vi "Artikeldaten_laden.vi"(8 "Fehler in":errorcluster, 11 "Cluster in":T1={"Initialisierung"={"Online?"=FALSE, "Grundpfad"=path "", "Kamera Oben"="", "IP-Adresse Flüssiglinse"="", "Flüssiglinse"=refnum, "Kamera Unten"="", "IP-Adresse SPS"="", "SPS-Verbindung"={"TCP Connection Ref"=refnum, "IP address"="", "timeout ms"=5000, "Connected?"=FALSE, "PLC Type"=enum."S7 1200", "Rack S7 400"=0, "Slot S7 400"=0, "PDU Size"=0, "connection semaphore"=refnum}, "IP-Adresse Lichtgitter"="", "Lichtgitter"=refnum, "Skalierungsfaktor"=0.0, "Bilder Oben"=[], "Bild Unten"=refnum, "Bild Ausschnitt Unten"=refnum}, "Einstellungen"={"Gesamtablauf gestartet"=FALSE, "i. O. Bilder speichern"=FALSE, "Bildspeicherung Offline"=FALSE, "Ausgewähltes Offline-Datum"="", "Ausgewähltes Offline-Teil"="", "Speicherpfad Bilder"=path ""}, "Artikeldaten"={"Artikelnummer"="", "Fertigungsauftrag"="", "Muster ISO"=refnum, "Belichtungszeit Referenzmarken"=0.0, "Fokus Referenzmarken"=0.0, "Belichtungszeit ISO"=0.0, "Fokus ISO"=0.0, "Belichtungszeit Unten"=0.0, "Kontaktanzahl"=0, "Aktueller Kontakt"=0, "Kontaktposition"={"x"=0.0, "y"=0.0}, "ISO-Muster nicht vorhanden"=FALSE, "Winkel ISO"=0.0, "Mittelpunkt ISO"={"x"=0.0, "y"=0.0}}, "Werte Kamera Oben"={"Koordinatensystem"={"Punkt x-Achse"={"X"=0.0, "Y"=0.0}, "Ursprung"={"X"=0.0, "Y"=0.0}, "Punkt y-Achse"={"X"=0.0, "Y"=0.0}}, "Position Kontakt"={"x"=0.0, "y"=0.0}, "Durchmesser Loch"=0.0, "Winkel Kontakt"=0.0, "Position Kontakt umgerechnet"={"x"=0.0, "y"=0.0}}, "Werte Kamera Unten"={"Prüfung Unten n. i. O."=FALSE}, "Werte Lichtgitter"={"Messwerte Referenzmarken"=[], "Mittelpunkt Referenzmarken"={"x"=0.0, "y"=0.0}, "Messwerte Kontakt"=[], "Offset"={"x"=0.0, "y"=0.0}}, "Rückmeldungen"={"Koordinaten ermittelt"=FALSE, "Vermessung Lichtgitter fertig"=FALSE, "Nachkontrolle Kamera Unten fertig"=FALSE}, "Fehler"={"Referenzen nicht gefunden"=FALSE, "Kontakt nicht gefunden"=FALSE, "Referenzen nicht in Lichtgitter"=FALSE, "Kontakt zu groß"=FALSE, "Kontakt zu klein"=FALSE}, "Statistik"={"Statistiken"=[]}, "Timer"={"Timer Start Position"=0, "Timer Start Lichtgitter"=0, "Timer Start Kamera Unten"=0}}) -> (0 "Fehler out":errorcluster, 1 "Anzahl Bilder out":i32, 2 "Offline Teile-Datum out":string[](array[string]), 3 "Cluster out":T1={"Initialisierung"={"Online?"=FALSE, "Grundpfad"=path "", "Kamera Oben"="", "IP-Adresse Flüssiglinse"="", "Flüssiglinse"=refnum, "Kamera Unten"="", "IP-Adresse SPS"="", "SPS-Verbindung"={"TCP Connection Ref"=refnum, "IP address"="", "timeout ms"=5000, "Connected?"=FALSE, "PLC Type"=enum."S7 1200", "Rack S7 400"=0, "Slot S7 400"=0, "PDU Size"=0, "connection semaphore"=refnum}, "IP-Adresse Lichtgitter"="", "Lichtgitter"=refnum, "Skalierungsfaktor"=0.0, "Bilder Oben"=[], "Bild Unten"=refnum, "Bild Ausschnitt Unten"=refnum}, "Einstellungen"={"Gesamtablauf gestartet"=FALSE, "i. O. Bilder speichern"=FALSE, "Bildspeicherung Offline"=FALSE, "Ausgewähltes Offline-Datum"="", "Ausgewähltes Offline-Teil"="", "Speicherpfad Bilder"=path ""}, "Artikeldaten"={"Artikelnummer"="", "Fertigungsauftrag"="", "Muster ISO"=refnum, "Belichtungszeit Referenzmarken"=0.0, "Fokus Referenzmarken"=0.0, "Belichtungszeit ISO"=0.0, "Fokus ISO"=0.0, "Belichtungszeit Unten"=0.0, "Kontaktanzahl"=0, "Aktueller Kontakt"=0, "Kontaktposition"={"x"=0.0, "y"=0.0}, "ISO-Muster nicht vorhanden"=FALSE, "Winkel ISO"=0.0, "Mittelpunkt ISO"={"x"=0.0, "y"=0.0}}, "Werte Kamera Oben"={"Koordinatensystem"={"Punkt x-Achse"={"X"=0.0, "Y"=0.0}, "Ursprung"={"X"=0.0, "Y"=0.0}, "Punkt y-Achse"={"X"=0.0, "Y"=0.0}}, "Position Kontakt"={"x"=0.0, "y"=0.0}, "Durchmesser Loch"=0.0, "Winkel Kontakt"=0.0, "Position Kontakt umgerechnet"={"x"=0.0, "y"=0.0}}, "Werte Kamera Unten"={"Prüfung Unten n. i. O."=FALSE}, "Werte Lichtgitter"={"Messwerte Referenzmarken"=[], "Mittelpunkt Referenzmarken"={"x"=0.0, "y"=0.0}, "Messwerte Kontakt"=[], "Offset"={"x"=0.0, "y"=0.0}}, "Rückmeldungen"={"Koordinaten ermittelt"=FALSE, "Vermessung Lichtgitter fertig"=FALSE, "Nachkontrolle Kamera Unten fertig"=FALSE}, "Fehler"={"Referenzen nicht gefunden"=FALSE, "Kontakt nicht gefunden"=FALSE, "Referenzen nicht in Lichtgitter"=FALSE, "Kontakt zu groß"=FALSE, "Kontakt zu klein"=FALSE}, "Statistik"={"Statistiken"=[]}, "Timer"={"Timer Start Position"=0, "Timer Start Lichtgitter"=0, "Timer Start Kamera Unten"=0}})   [LabVIEW 2024]
doc: "Lädt die Artikeldaten aus den Globalen Variablen, bzw. im \"Offline-Modus\" aus der Konfig Datei in das Cluster."
uses:
  Typdefinitionen/Cluster.ctl
  <vilib>/userDefined/High Color/IMAQdx.ctl
  <vilib>/DATA AHEAD/SP7/typedefs/S7 Connection.ctl
  <vilib>/DATA AHEAD/SP7/typedefs/PLC Type.ctl
  <vilib>/vision/Image Controls.llb/IMAQ Image.ctl
  Typdefinitionen/Koordinatensystem.ctl
  Typdefinitionen/Statistik.ctl
  <vilib>/Utility/config.llb/Read Key (U32).vi
  <vilib>/Utility/config.llb/Read Key (Double).vi
  Sonstige/Globale Variablen.vi
  <vilib>/Utility/config.llb/Write Key (U32).vi
  <vilib>/Utility/config.llb/Write Key (Double).vi
  <vilib>/Utility/config.llb/NI_LVConfig.lvlib
  <vilib>/DATA AHEAD/SP7/SP7.lvlib
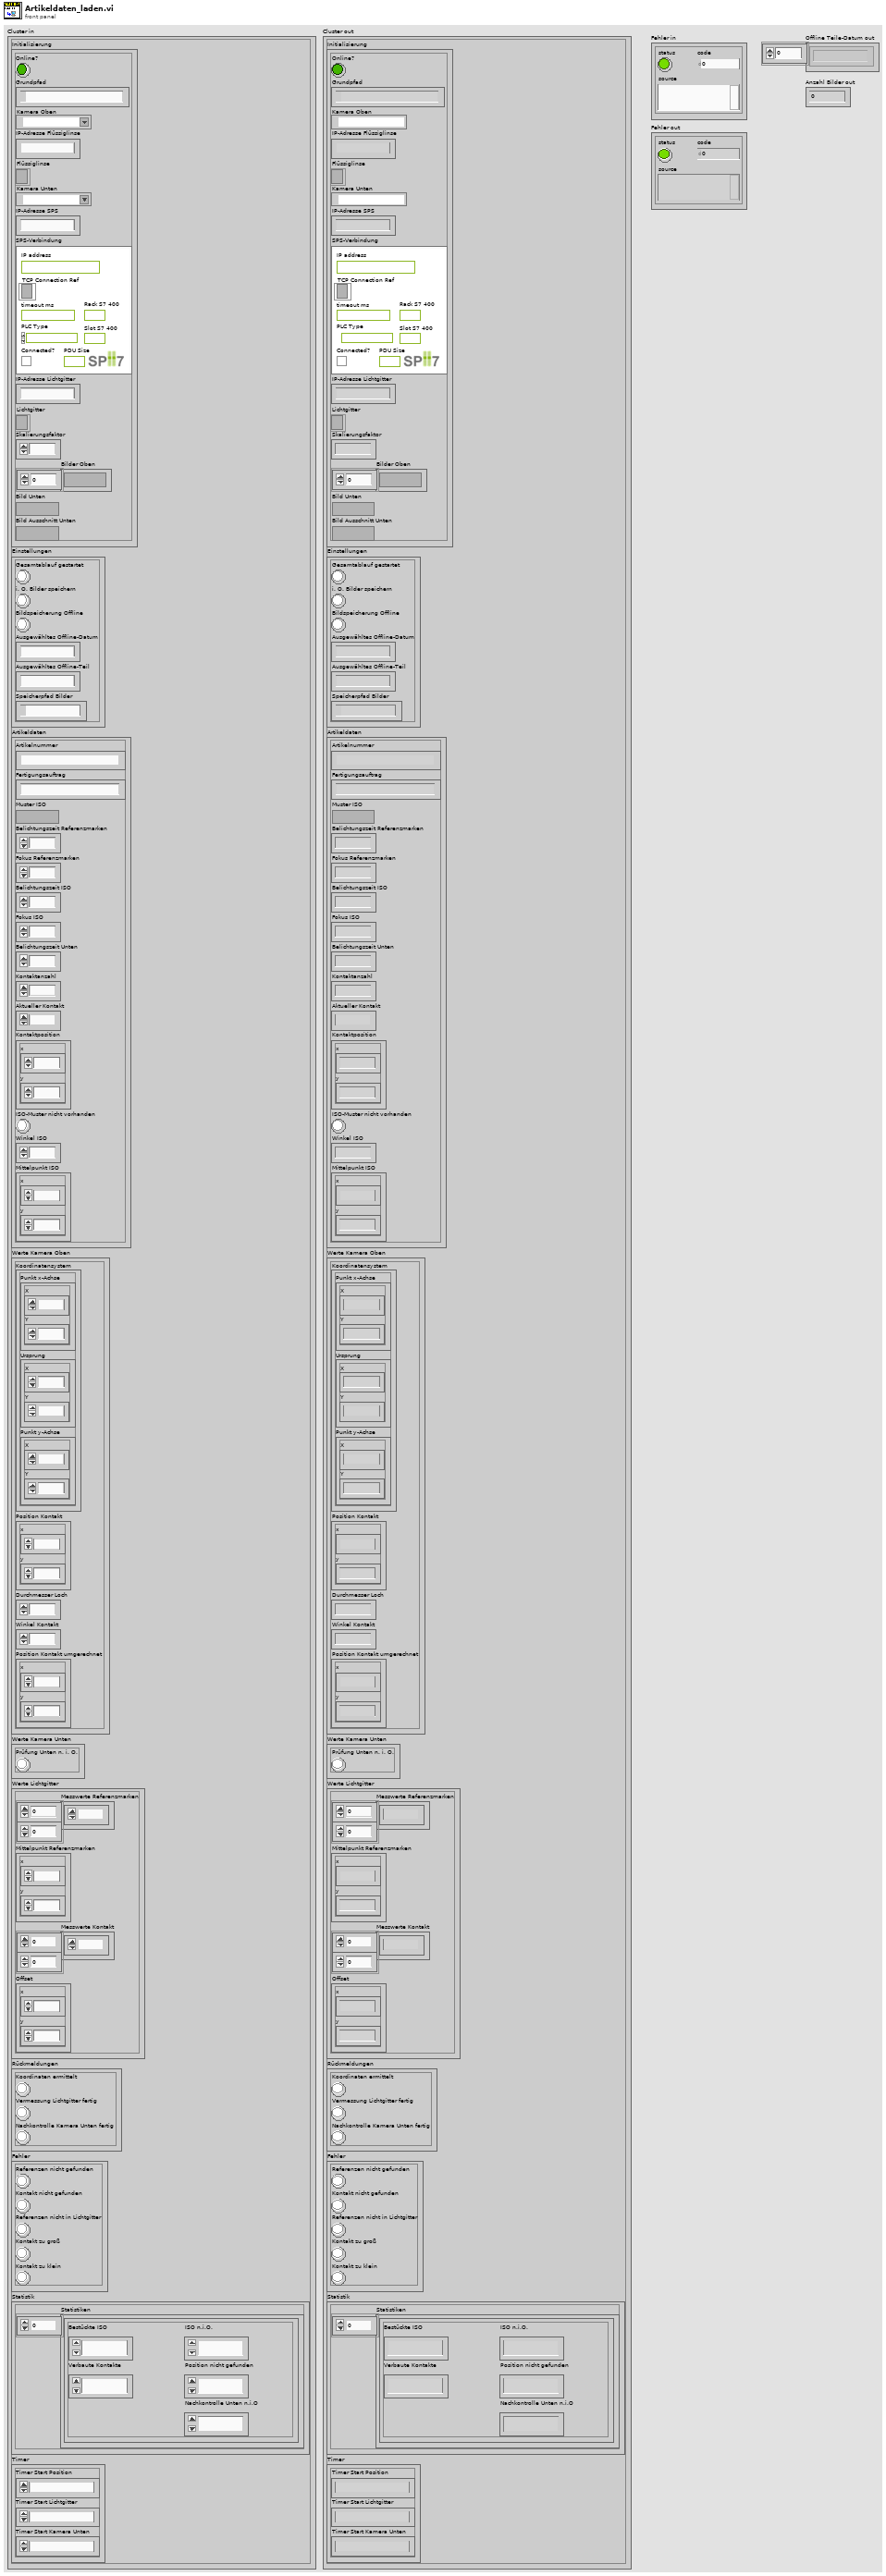
[diagram p1: front panel]
types:
  T1 = typedef "Cluster.ctl" = cluster{"Initialisierung":cluster{"Online?":bool, "Grundpfad":path, "Kamera Oben":T2, "IP-Adresse Flüssiglinse":string, "Flüssiglinse":refnum<k5>, "Kamera Unten":T2, "IP-Adresse SPS":string, "SPS-Verbindung":T3, "IP-Adresse Lichtgitter":string, "Lichtgitter":refnum<k5>, "Skalierungsfaktor":dbl, "Bilder Oben":T6[], "Bild Unten":T6, "Bild Ausschnitt Unten":T6}, "Einstellungen":cluster{"Gesamtablauf gestartet":bool, "i. O. Bilder speichern":bool, "Bildspeicherung Offline":bool, "Ausgewähltes Offline-Datum":string, "Ausgewähltes Offline-Teil":string, "Speicherpfad Bilder":path}, "Artikeldaten":cluster{"Artikelnummer":string, "Fertigungsauftrag":string, "Muster ISO":T6, "Belichtungszeit Referenzmarken":dbl, "Fokus Referenzmarken":dbl, "Belichtungszeit ISO":dbl, "Fokus ISO":dbl, "Belichtungszeit Unten":dbl, "Kontaktanzahl":u32, "Aktueller Kontakt":i16, "Kontaktposition":cluster{"x":sgl, "y":sgl}, "ISO-Muster nicht vorhanden":bool, "Winkel ISO":sgl, "Mittelpunkt ISO":cluster{"x":dbl, "y":dbl}}, "Werte Kamera Oben":cluster{"Koordinatensystem":T7, "Position Kontakt":cluster{"x":dbl, "y":dbl}, "Durchmesser Loch":dbl, "Winkel Kontakt":dbl, "Position Kontakt umgerechnet":cluster{"x":dbl, "y":dbl}}, "Werte Kamera Unten":cluster{"Prüfung Unten n. i. O.":bool}, "Werte Lichtgitter":cluster{"Messwerte Referenzmarken":dbl[][], "Mittelpunkt Referenzmarken":cluster{"x":dbl, "y":dbl}, "Messwerte Kontakt":dbl[][], "Offset":cluster{"x":dbl, "y":dbl}}, "Rückmeldungen":cluster{"Koordinaten ermittelt":bool, "Vermessung Lichtgitter fertig":bool, "Nachkontrolle Kamera Unten fertig":bool}, "Fehler":cluster{"Referenzen nicht gefunden":bool, "Kontakt nicht gefunden":bool, "Referenzen nicht in Lichtgitter":bool, "Kontakt zu groß":bool, "Kontakt zu klein":bool}, "Statistik":cluster{"Statistiken":T8[]}, "Timer":cluster{"Timer Start Position":u32, "Timer Start Lichtgitter":u32, "Timer Start Kamera Unten":u32}}
  T2 = typedef "IMAQdx.ctl" = refnum<k21>
  T3 = typedef "SP7.lvlib/S7 Connection.ctl" = cluster{"TCP Connection Ref":refnum<k5>, "IP address":string, "timeout ms":i32, "Connected?":bool, "PLC Type":T4, "Rack S7 400":u8, "Slot S7 400":u8, "PDU Size":u16, "connection semaphore":T5}
  T4 = typedef "SP7.lvlib/PLC Type.ctl" = enum16{"S7 200", "S7 300/400", "S7 1200", "S7 1500", "LOGO!8"}
  T5 = typedef "Semaphore RefNum" = refnum<k1>
  T6 = typedef "IMAQ Image.ctl" = refnum<image>
  T7 = typedef "Koordinatensystem.ctl" = cluster{"Punkt x-Achse":cluster{"X":sgl, "Y":sgl}, "Ursprung":cluster{"X":sgl, "Y":sgl}, "Punkt y-Achse":cluster{"X":sgl, "Y":sgl}}
  T8 = typedef "Statistik.ctl" = cluster{"Bestückte ISO":u32, "Verbaute Kontakte":u32, "ISO n.i.O.":u32, "Nachkontrolle Unten n.i.O":u32, "Position nicht gefunden":u32}
  T9 = typedef "NI_LVConfig.lvlib/Config Data RefNum.ctl" = refnum<k1>
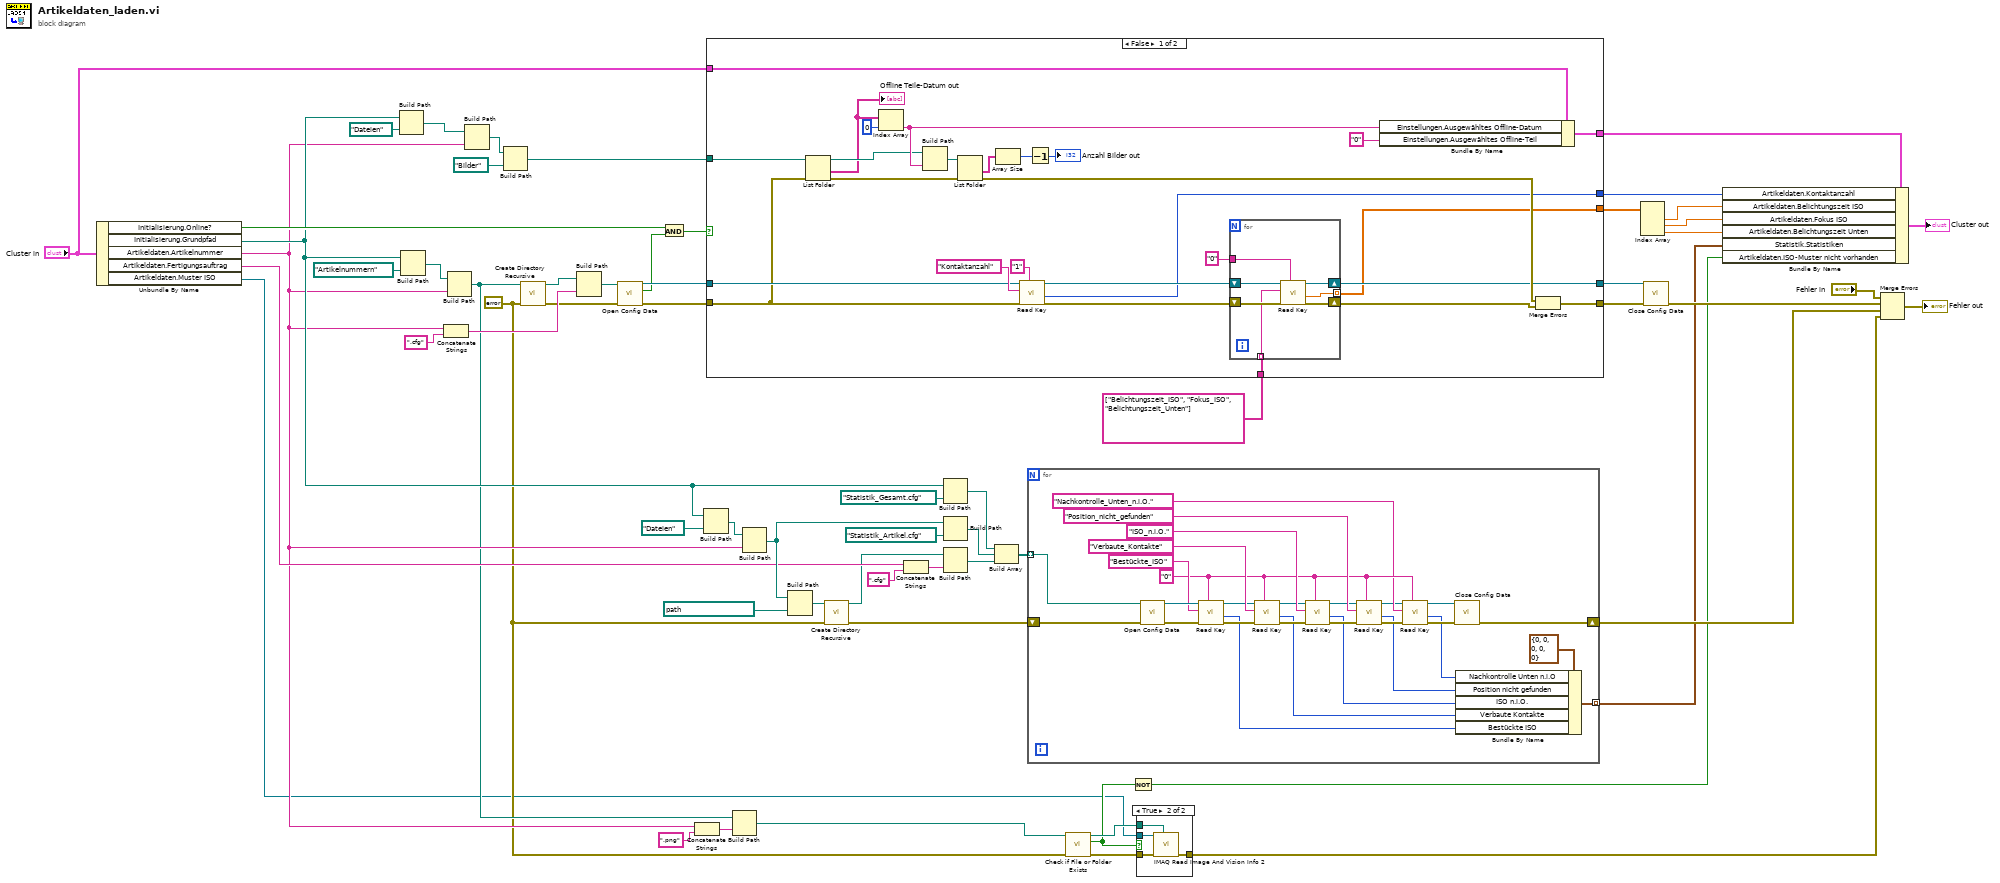
[diagram p0: block diagram]
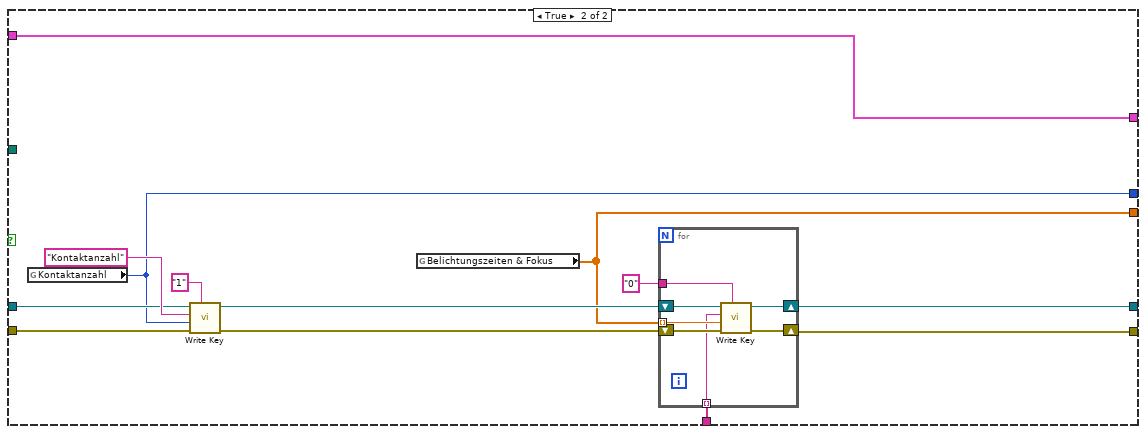
[diagram p2: hidden frame]
diagram:
  w5 = errorcluster {"status"=FALSE, "code"=0, "source"=""} ("error in (no error)")
  n1 = Unbundle By Name("Cluster in") -> ("Initialisierung.Online?"=w29:bool, "Initialisierung.Grundpfad"=w14:path, "Artikeldaten.Artikelnummer"=w10:string, "Artikeldaten.Fertigungsauftrag"=w32:string, "Artikeldaten.Muster ISO"=w1:T6)
  n2 = Build Path(base path=w14, name or relative path=path "Dateien") -> (appended path=w24:path)
  n3 = Build Path(base path=w14, name or relative path=path "Artikelnummern") -> (appended path=w60:path)
  n4 = Concatenate Strings(w10, ".cfg" ("string")) -> (w58:string)
  n5 = Build Path(base path=w60, name or relative path=w10) -> (appended path=w9:path)
  n6 = Build Path(base path=w24, name or relative path=w10) -> (appended path=w27:path)
  n7 = Build Path(base path=w27, name or relative path=path "Bilder") -> (appended path=w26:path)
  n8 = call <vilib>:"Create Directory Recursive.vi"("error in (no error)"=w5, "directory"=w9) -> ("error out"=w22:errorcluster, "directory copy"=w21:path)  [unwired: 3 in, 1 out]
  n9 = Build Path(base path=w21, name or relative path=w58) -> (appended path=w57:path)
  n10 = call <vilib>:"Open Config Data.vi"("error in (no error)"=w22, "configuration file path"=w57) -> ("error out"=w55:errorcluster, "file created?"=w13:bool, "refnum"=w56:T9)  [unwired: 7 in]
  n11 = And(x=w29, y=w13) -> (x .and. y?=w28:bool)
  n12 = Concatenate Strings(w10, ".png" ("string")) -> (w11:string)
  n13 = Build Path(base path=w14, name or relative path=path "Dateien") -> (appended path=w42:path)
  n14 = case shown="False" w28 {
    tunnel: w56 -> [w88 w108]
    tunnel: w55 -> [w74 w107]
    tunnel: [w66 w102] -> w54
    tunnel: [w72 w101] -> w53
    tunnel: [w71 w99] -> w47
    tunnel: "Cluster in" -> [w70 w99]
    tunnel: string[] ["Belichtungszeit_ISO", "Fokus_ISO", "Belichtungszeit_Unten"] -> [w69 w100]
    tunnel: [w65 w97] -> w46
    tunnel: [w64 w98] -> w45
    tunnel: w26 -> [w63 _]
    frame False {
      n15 = List Folder(path=w63, error in=w74) -> (path out=w80:path, folder names=w77:string[], error out=w83:errorcluster)  [unwired: 2 in, 1 out]
      "Offline Teile-Datum out" <- w77
      n16 = Index Array(array=w77, index=0) -> (element=w81:string)
      n17 = Build Path(base path=w80, name or relative path=w81) -> (appended path=w82:path)
      n18 = List Folder(path=w82, error in=w83) -> (folder names=w84:string[], error out=w73:errorcluster)  [unwired: 2 in, 2 out]
      n19 = Array Size(array=w84) -> (size(s)=w78:i32)
      n20 = call-poly <vilib>:"Read Key.vi"("section"="1", "error in (no error)"=w74, "key"="Kontaktanzahl", "refnum"=w88) -> ("error out"=w87:errorcluster, "value"=w65:u32, "refnum out"=w86:T9)  [unwired: 4 in, 1 out]
      n21 = Decrement(x=w78) -> (x-1=→"Anzahl Bilder out":i32)
      n22 = for {
        shift-right: [w92] -> w66
        shift-left: w86 -> [w95]
        shift-right: [w91] -> w67
        shift-left: w87 -> [w96]
        tunnel: w69 -> [w94] mode=indexing
        tunnel: "0" ("section") -> [w93]
        tunnel: [w90] -> w64 mode=indexing
        n23 = call-poly <vilib>:"Read Key.vi"("section"=w93, "error in (no error)"=w96, "key"=w94, "refnum"=w95) -> ("error out"=w91:errorcluster, "value"=w90:dbl, "refnum out"=w92:T9)  [unwired: 4 in, 1 out]
      }
      n24 = Bundle By Name(cluster=w70, "Einstellungen.Ausgewähltes Offline-Datum"=w81, "Einstellungen.Ausgewähltes Offline-Teil"="0") -> (w71:T1)
      n25 = Merge Errors(w73, w67) -> (w72:errorcluster)
    }
    frame True {
      n26 = global read "Globale Variablen.vi" "Kontaktanzahl"() -> (w97:u32)
      n27 = call-poly <vilib>:"Write Key.vi"("section"="1", "error in (no error)"=w107, "value"=w97, "key"="Kontaktanzahl", "refnum"=w108) -> ("error out"=w105:errorcluster, "refnum out"=w106:T9)  [unwired: 4 in, 1 out]
      n28 = global read "Globale Variablen.vi" "Belichtungszeiten & Fokus"() -> (w98:dbl[])
      n29 = for {
        shift-right: [w113] -> w102
        shift-left: w106 -> [w116]
        shift-right: [w112] -> w101
        shift-left: w105 -> [w115]
        tunnel: "0" ("section") -> [w114]
        tunnel: w98 -> [w111] mode=indexing
        tunnel: w100 -> [w110] mode=indexing
        n30 = call-poly <vilib>:"Write Key.vi"("section"=w114, "error in (no error)"=w115, "value"=w111, "key"=w110, "refnum"=w116) -> ("error out"=w112:errorcluster, "refnum out"=w113:T9)  [unwired: 4 in, 1 out]
      }
    }
  }
  n31 = Build Path(base path=w9, name or relative path=w11) -> (appended path=w6:path)
  n32 = Build Path(base path=w42, name or relative path=w10) -> (appended path=w38:path)
  n33 = Build Path(base path=w38, name or relative path=path "Fertigungsaufträge") -> (appended path=w19:path)
  n34 = call <vilib>:"Create Directory Recursive.vi"("error in (no error)"=w5, "directory"=w19) -> ("error out"=w17:errorcluster, "directory copy"=w18:path)  [unwired: 3 in, 1 out]
  n35 = Concatenate Strings(w32, ".cfg" ("string")) -> (w33:string)
  n36 = Build Path(base path=w14, name or relative path=path "Statistik_Gesamt.cfg") -> (appended path=w39:path)
  n37 = Build Path(base path=w38, name or relative path=path "Statistik_Artikel.cfg") -> (appended path=w36:path)
  n38 = Build Path(base path=w18, name or relative path=w33) -> (appended path=w20:path)
  n39 = Build Array(w39, w36, w20) -> (w35:path[])
  n40 = for {
    shift-right: [w126] -> w31
    shift-left: w17 -> [w125]
    tunnel: w35 -> [w124] mode=indexing
    tunnel: [w117] -> w30 mode=indexing
    w134 = "0" ("section")
    n41 = call <vilib>:"Open Config Data.vi"("error in (no error)"=w125, "configuration file path"=w124) -> ("error out"=w141:errorcluster, "refnum"=w144:T9)  [unwired: 7 in, 1 out]
    n42 = call-poly <vilib>:"Read Key.vi"("section"=w134, "error in (no error)"=w141, "key"="Bestückte_ISO", "refnum"=w144) -> ("error out"=w142:errorcluster, "value"=w122:u32, "refnum out"=w127:T9)  [unwired: 4 in, 1 out]
    n43 = call-poly <vilib>:"Read Key.vi"("section"=w134, "error in (no error)"=w142, "key"="Verbaute_Kontakte", "refnum"=w127) -> ("error out"=w140:errorcluster, "value"=w121:u32, "refnum out"=w128:T9)  [unwired: 4 in, 1 out]
    n44 = call-poly <vilib>:"Read Key.vi"("section"=w134, "error in (no error)"=w140, "key"="ISO_n.i.O.", "refnum"=w128) -> ("error out"=w139:errorcluster, "value"=w120:u32, "refnum out"=w129:T9)  [unwired: 4 in, 1 out]
    n45 = call-poly <vilib>:"Read Key.vi"("section"=w134, "error in (no error)"=w139, "key"="Position_nicht_gefunden", "refnum"=w129) -> ("error out"=w138:errorcluster, "value"=w119:u32, "refnum out"=w130:T9)  [unwired: 4 in, 1 out]
    n46 = call-poly <vilib>:"Read Key.vi"("section"=w134, "error in (no error)"=w138, "key"="Nachkontrolle_Unten_n.i.O.", "refnum"=w130) -> ("error out"=w132:errorcluster, "value"=w118:u32, "refnum out"=w131:T9)  [unwired: 4 in, 1 out]
    n47 = call <vilib>:"Close Config Data.vi"("error in (no error)"=w132, "refnum"=w131) -> ("error out"=w126:errorcluster)  [unwired: 8 in, 1 out]
    n48 = Bundle By Name(cluster=T8 {"Bestückte ISO"=0, "Verbaute Kontakte"=0, "ISO n.i.O."=0, "Nachkontrolle Unten n.i.O"=0, "Position nicht gefunden"=0} ("Cluster"), "Nachkontrolle Unten n.i.O"=w118, "Position nicht gefunden"=w119, "ISO n.i.O."=w120, "Verbaute Kontakte"=w121, "Bestückte ISO"=w122) -> (w117:T8)
  }
  n49 = call <vilib>:"Check if File or Folder Exists.vi"("error in (no error)"=w5, "path"=w6) -> ("error out"=w8:errorcluster, "file or folder exists?"=w3:bool, "dup path"=w7:path)  [unwired: 7 in]
  n50 = Not(x=w3) -> (.not. x?=w2:bool)
  n51 = case shown="True" w3 {
    tunnel: [w145 w149] -> w4
    tunnel: w8 -> [w145 w148]
    tunnel: w7 -> [_ w147]
    tunnel: w1 -> [_ w146]
    frame False {
    }
    frame True {
      n52 = call "IMAQ Read Image And Vision Info 2"("File Path"=w147, "error in (no error)"=w148, "Image"=w146) -> ("error out"=w149:errorcluster)  [unwired: 6 in, 2 out]
    }
  }
  n53 = Index Array(array=w45) -> (element #1=w48:dbl, element #2=w16:dbl, element #3=w15:dbl)  [unwired: 3 in]
  n54 = call <vilib>:"Close Config Data.vi"("error in (no error)"=w53, "refnum"=w54) -> ("error out"=w50:errorcluster)  [unwired: 8 in, 1 out]
  n55 = Bundle By Name(cluster=w47, "Artikeldaten.Kontaktanzahl"=w46, "Artikeldaten.Belichtungszeit ISO"=w48, "Artikeldaten.Fokus ISO"=w16, "Artikeldaten.Belichtungszeit Unten"=w15, "Statistik.Statistiken"=w30, "Artikeldaten.ISO-Muster nicht vorhanden"=w2) -> (→"Cluster out":T1)
  n56 = Merge Errors("Fehler in", w50, w31, w4) -> (→"Fehler out":errorcluster)
